vi "Dispose_lc.vi"(8 "error in (no error)":errorcluster caption="错误输入（无错误）", 11 "Picture_Class 输入":refnum<class "Picture_Class.lvclass"> caption="DNL_LabVIEW Object in") -> (0 "error out":errorcluster caption="错误输出", 3 "Picture_Class 输出":refnum<class "Picture_Class.lvclass"> caption="DNL_LabVIEW Object out")   [LabVIEW 2013, in "Picture_Class.lvclass"]
uses:
  Picture_Class.lvclass
  Picture_Class.lvclass/Picture_Class.ctl
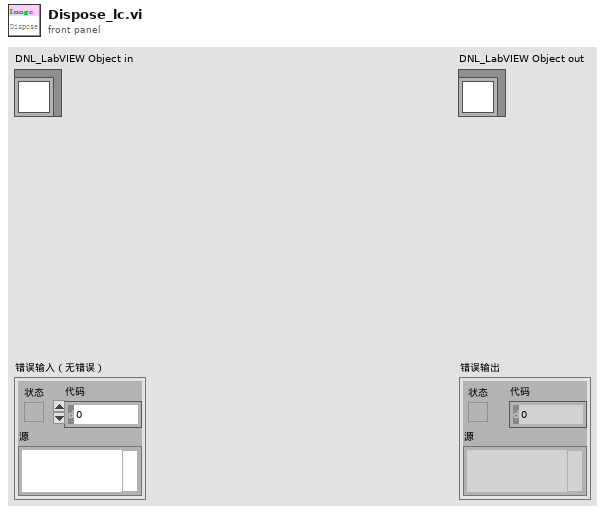
[diagram p1: front panel]
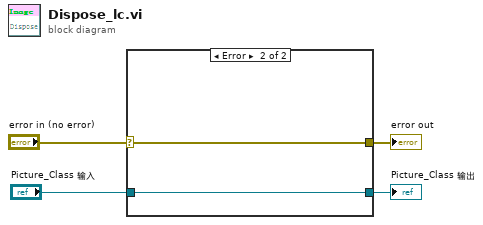
[diagram p0: block diagram]
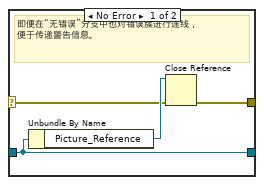
[diagram p2: hidden frame]
diagram:
  n1 = case shown="Error" "error in (no error)" {
    selector: "error in (no error)" -> [w6 w10]
    tunnel: [w5 w10] -> w3
    tunnel: [w8 w9] -> w1
    tunnel: "Picture_Class 输入" -> [w8 w9]
    frame No Error {
      # "即便在“无错误”分支中也对错误簇进行连线，\n便于传递警告信息。"
      n2 = Unbundle By Name(w8) -> ("Picture_Reference"=w7:refnum<vi>)
      n3 = Close Reference(reference=w7, error in (no error)=w6) -> (error out=w5:errorcluster)
    }
    frame Error {
    }
  }
  "error out" <- w3
  "Picture_Class 输出" <- w1
